vi "Demo.vi"() -> ()   [LabVIEW 2018]
doc: "本VI是为《我和LabVIEW》一书编写的示例。\n关于本书的介绍请参考网页：\nhttp://ruanqizhen.spaces.live.com/blog/cns!5852D4F797C53FB6!4310.entry"
uses:
  Othello.xctl
panel:
  out "messege":string
  in  "new":bool
  in  "exit":bool
  in  "Othello":T1[][](xcontrol)
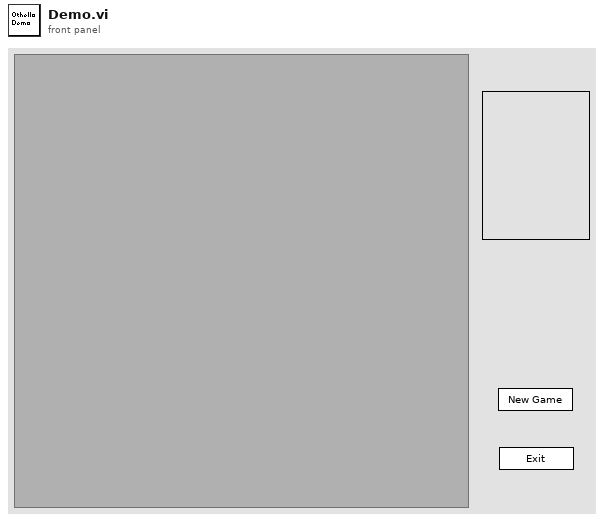
[diagram p1: front panel]
types:
  T1 = typedef "Othello.xctl/Pict Ring Chess.ctl" = u16
  T2 = typedef "Othello.xctl/Interactive Action.ctl" = refnum<user-event>
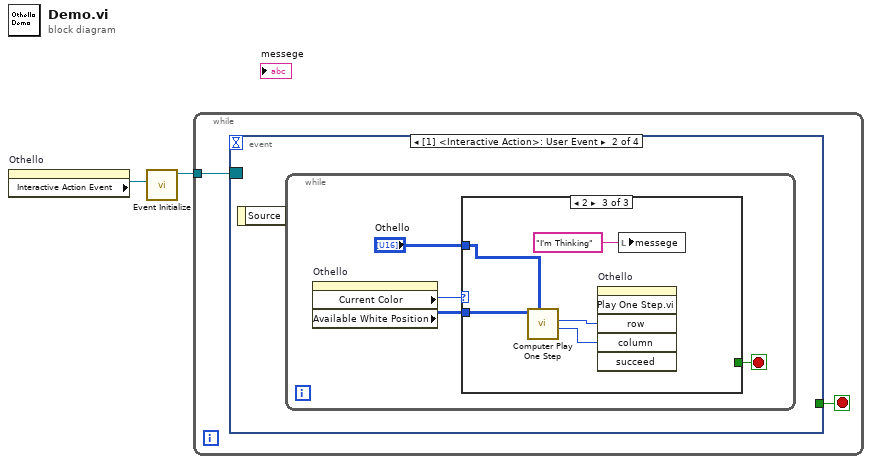
[diagram p0: block diagram]
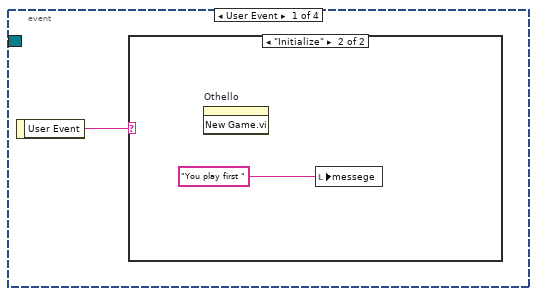
[diagram p2: hidden frame]
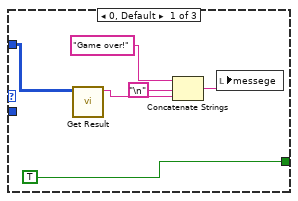
[diagram p4: hidden frame]
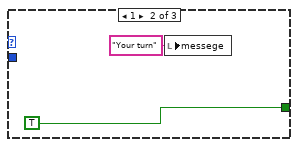
[diagram p5: hidden frame]
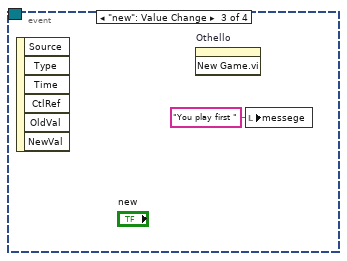
[diagram p6: hidden frame]
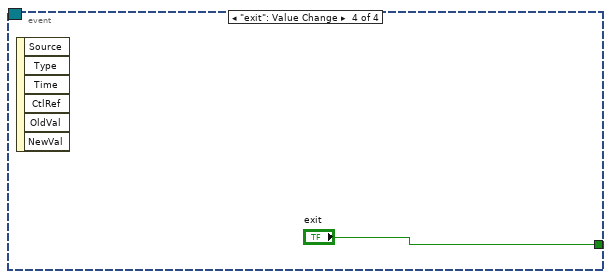
[diagram p7: hidden frame]
diagram:
  n1 = property on="Othello" class="Othello (strict)"() -> ("Interactive Action Event"=w1:T2)  [unwired: 2 in, 2 out]
  n2 = call "Event Initialize.vi"("Interactive Action"=w1) -> ("Event Reg Ref"=w2:refnum<event-registration>)  [unwired: 10 out]
  n3 = while {
    tunnel: w2 -> [w4]
    stop <- w3 stop-if-true
    n4 = event shown="[1] <Interactive Action>: User Event" {
      selector: w4 -> [_ _ _ _]
      dyn-events: _ -> [_ _ _ _]
      timeout: _ -> [_ _ _ _]
      tunnel: [_ _ _ "exit"] -> w3
      event User Event {
        n5 = event-data() -> ("User Event"=w5:string)  [unwired: 1 out]
        n6 = case shown="\"Initialize\"" w5 {
          frame "假", Default {
          }
          frame "Initialize" {
            n7 = invoke on="Othello" class="Othello (严格)" method="New Game.vi"() -> ()  [unwired: 3 in, 3 out]
            n8 = local write "messege"("You play first " ("messege")) -> ()
          }
        }
      }
      event User Event {
        n9 = event-data() -> ()  [unwired: 2 out]
        n10 = while {
          stop <- w9 stop-if-true
          n11 = property on="Othello" class="Othello (strict)"() -> ("Current Color"=w10:T1, "Available White Position"=w8:i32[][])  [unwired: 2 in, 2 out]
          n12 = case shown="2" w10 {
            tunnel: [TRUE TRUE _] -> w9
            tunnel: w8 -> [_ _ w22]
            tunnel: "Othello" -> [w11 _ w19]
            frame 0, Default {
              n13 = call "Get Result.vi"("Othello"=w11) -> ("Resule"=w15:string)  [unwired: 10 out]
              n14 = Concatenate Strings("Game over!" ("messege"), "\n", w15) -> (w13:string)
              n15 = local write "messege"(w13) -> ()
            }
            frame 1 {
              n16 = local write "messege"("Your turn" ("messege")) -> ()
            }
            frame 2 {
              n17 = call "Computer Play One Step.vi"("board"=w19, "Available White Position"=w22) -> ("column"=w20:i32, "row"=w21:i32)  [unwired: 1 in, 7 out]
              n18 = invoke on="Othello" class="Othello (严格)" method="Play One Step.vi"("row"=w21, "column"=w20) -> ()  [unwired: 4 in, 6 out]
              n19 = local write "messege"("I'm Thinking" ("messege")) -> ()
            }
          }
        }
      }
      event "new": Value Change {
        n20 = event-data() -> ()  [unwired: 7 out]
        n21 = invoke on="Othello" class="Othello (严格)" method="New Game.vi"() -> ()  [unwired: 3 in, 3 out]
        n22 = local write "messege"("You play first " ("messege")) -> ()
      }
      event "exit": Value Change {
        n23 = event-data() -> ()  [unwired: 7 out]
      }
    }
  }
